vi "Comparison Operations with CASE S.vi"() -> ()   [LabVIEW 2020]
panel:
  in  "COMPARISON":string
  in  "y":dbl
  in  "x":dbl
  out "RESULT":bool
  out "Boolean":bool
  in  "X":dbl
  in  "Y":dbl
  # "COMPARISON OPs WITH CASE STRUCTURE"
  # "COMPARISONS:\nx=y?\nx=/y?\nx=0?\nx=/0?\ny=0?\ny=/0?\nx>y?\nx<y?\nx>0?\ny>0?\ny<0?\nx<0?\nx>=0?\nx<=0?\ny>=0?\ny<=0?\nx>=y?\nx<=y?"
  # "DDS"
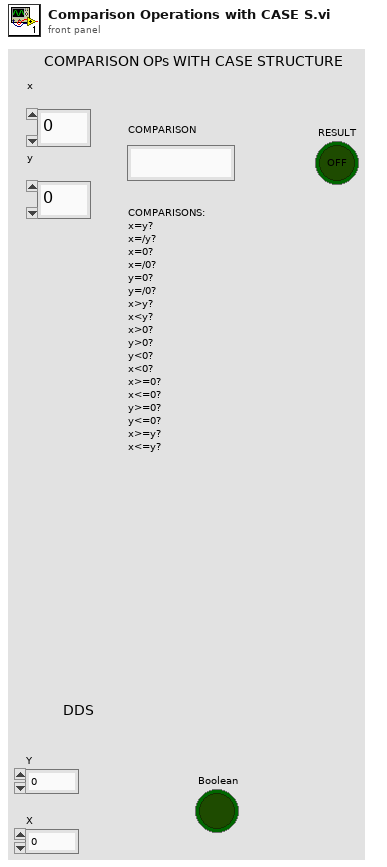
[diagram p1: front panel]
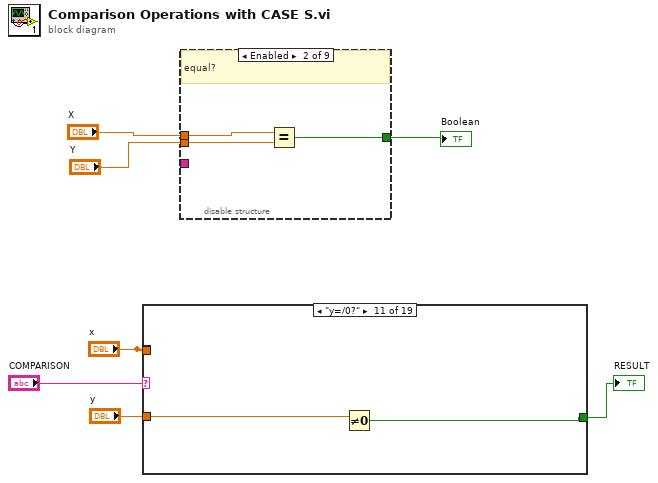
[diagram p0: block diagram]
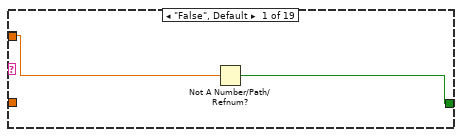
[diagram p2: hidden frame]
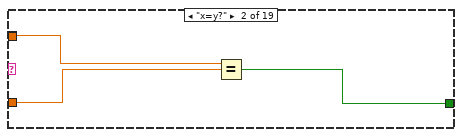
[diagram p3: hidden frame]
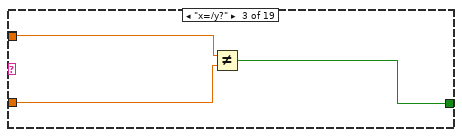
[diagram p4: hidden frame]
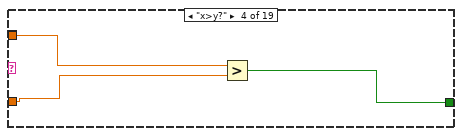
[diagram p5: hidden frame]
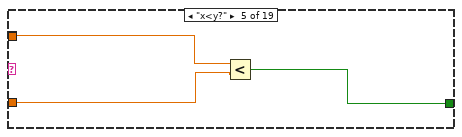
[diagram p6: hidden frame]
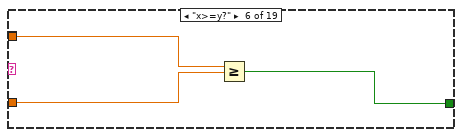
[diagram p7: hidden frame]
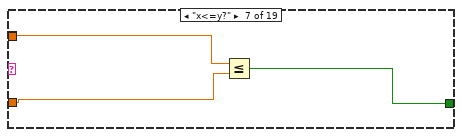
[diagram p8: hidden frame]
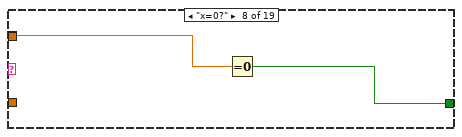
[diagram p9: hidden frame]
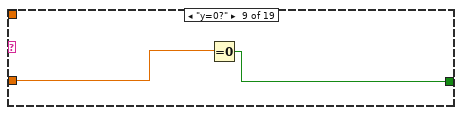
[diagram p10: hidden frame]
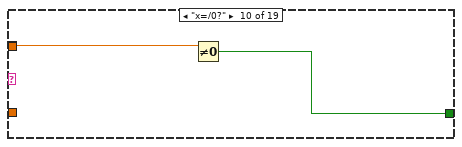
[diagram p11: hidden frame]
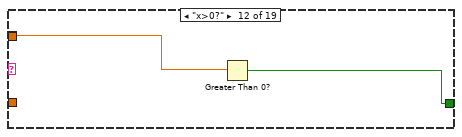
[diagram p12: hidden frame]
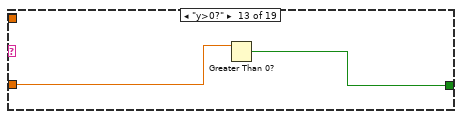
[diagram p13: hidden frame]
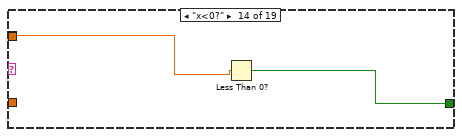
[diagram p14: hidden frame]
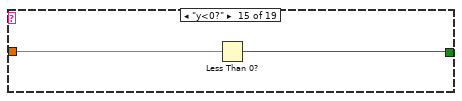
[diagram p15: hidden frame]
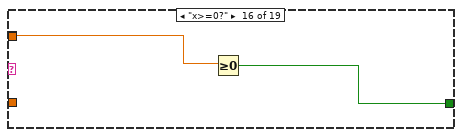
[diagram p16: hidden frame]
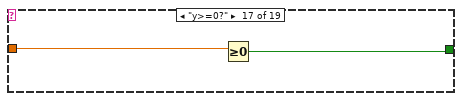
[diagram p17: hidden frame]
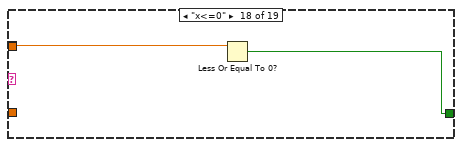
[diagram p18: hidden frame]
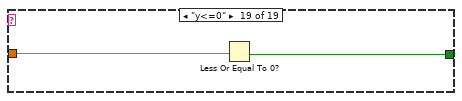
[diagram p19: hidden frame]
diagram:
  n1 = case shown="\"y=/0?\"" "COMPARISON" {
    tunnel: "x" -> [w10 w13 w16 _ w22 w25 w28 w30 _ w34 _ w38 _ w42 _ w46 _ w50 _]
    tunnel: "y" -> [_ w12 w15 w18 w21 w24 w27 _ w32 _ w36 _ w40 _ w44 _ w48 _ w52]
    tunnel: [w9 w11 w14 w17 w20 w23 w26 w29 w31 w33 w35 w37 w39 w41 w43 w45 w47 w49 w51] -> w2
    tunnel: "x" -> [_ _ _ w19 _ _ _ _ _ _ _ _ _ _ _ _ _ _ _]
    frame "False", Default {
      n2 = Not A Number/Path/Refnum?(number/path/refnum=w10) -> (NaN/Path/Refnum?=w9:bool)
    }
    frame "x=y?" {
      n3 = Equal?(x=w13, y=w12) -> (x = y?=w11:bool)
    }
    frame "x=/y?" {
      n4 = Not Equal?(x=w16, y=w15) -> (x != y?=w14:bool)
    }
    frame "x>y?" {
      n5 = Greater?(x=w19, y=w18) -> (0:w17:bool)
    }
    frame "x<y?" {
      n6 = Less?(x=w22, y=w21) -> (x < y?=w20:bool)
    }
    frame "x>=y?" {
      n7 = Greater Or Equal?(x=w25, y=w24) -> (x >= y?=w23:bool)
    }
    frame "x<=y?" {
      n8 = Less Or Equal?(x=w28, y=w27) -> (x <= y?=w26:bool)
    }
    frame "x=0?" {
      n9 = Equal To 0?(x=w30) -> (x = 0?=w29:bool)
    }
    frame "y=0?" {
      n10 = Equal To 0?(x=w32) -> (x = 0?=w31:bool)
    }
    frame "x=/0?" {
      n11 = Not Equal To 0?(x=w34) -> (x != 0?=w33:bool)
    }
    frame "y=/0?" {
      n12 = Not Equal To 0?(x=w36) -> (x != 0?=w35:bool)
    }
    frame "x>0?" {
      n13 = Greater Than 0?(x=w38) -> (x > 0?=w37:bool)
    }
    frame "y>0?" {
      n14 = Greater Than 0?(x=w40) -> (x > 0?=w39:bool)
    }
    frame "x<0?" {
      n15 = Less Than 0?(x=w42) -> (x < 0?=w41:bool)
    }
    frame "y<0?" {
      n16 = Less Than 0?(x=w44) -> (x < 0?=w43:bool)
    }
    frame "x>=0?" {
      n17 = Greater Or Equal To 0?(x=w46) -> (x >= 0?=w45:bool)
    }
    frame "y>=0?" {
      n18 = Greater Or Equal To 0?(x=w48) -> (x >= 0?=w47:bool)
    }
    frame "x<=0" {
      n19 = Less Or Equal To 0?(x=w50) -> (x <= 0?=w49:bool)
    }
    frame "y<=0" {
      n20 = Less Or Equal To 0?(x=w52) -> (x <= 0?=w51:bool)
    }
  }
  "RESULT" <- w2
  n21 = disable-structure "Diagram Disable Structure" shown="Enabled" {
    disable-tunnel: "Y" -> [_ w55 w58 w59 w63 w66 w69 w72 _]
    disable-tunnel: "X" -> [_ w54 w57 w60 w64 w67 w70 w73 w75]
    disable-tunnel: [_ w53 w56 w61 w62 w65 w68 w71 w74] -> w5
    disable-tunnel: [_ _ _ _ _ _ _ _ _] -> w6
    frame Disabled {
    }
    frame Enabled {
      # "equal?"
      n22 = Equal?(x=w54, y=w55) -> (x = y?=w53:bool)
    }
    frame Disabled {
      # "x equal to y?"
      n23 = Equal?(x=w57, y=w58) -> (x = y?=w56:bool)
    }
    frame Disabled {
      # "Not equal?"
      n24 = Not Equal?(x=w60, y=w59) -> (x != y?=w61:bool)
    }
    frame Disabled {
      # "x Greater than y?"
      n25 = Greater?(x=w64, y=w63) -> (0:w62:bool)
    }
    frame Disabled {
      # "x less than y?"
      n26 = Less?(x=w67, y=w66) -> (x < y?=w65:bool)
    }
    frame Disabled {
      # "x greater than or equal to y?"
      n27 = Greater Or Equal?(x=w70, y=w69) -> (x >= y?=w68:bool)
    }
    frame Disabled {
      # "x less then or equal to y?"
      n28 = Less Or Equal?(x=w73, y=w72) -> (x <= y?=w71:bool)
    }
    frame Disabled {
      # "x equal to 0?"
      n29 = Equal To 0?(x=w75) -> (x = 0?=w74:bool)
    }
  }
  "Boolean" <- w5
